vi "While_Factorial.vi"() -> ()   [LabVIEW 2024]
panel:
  out "Numeric 2":i32
  in  "Numeric":dbl
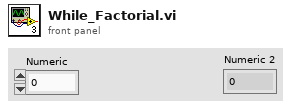
[diagram p1: front panel]
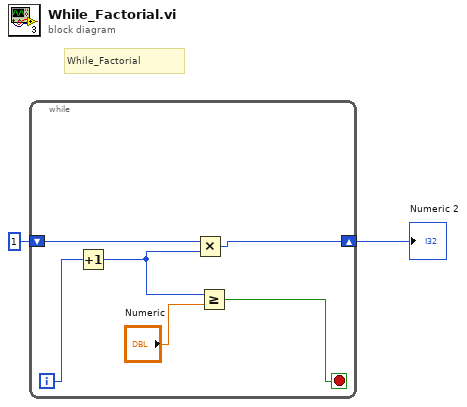
[diagram p0: block diagram]
diagram:
  # "While_Factorial"
  n1 = while {
    shift-right: [w6] -> w2
    shift-left: 1 -> [w3]
    i -> [w5]
    stop <- w8 stop-if-true
    n2 = Increment(x=w5) -> (x+1=w4:i32)
    n3 = Multiply(x=w3, y=w4) -> (x*y=w6:i32)
    n4 = Greater Or Equal?(x=w4, y="Numeric") -> (x >= y?=w8:bool)
  }
  "Numeric 2" <- w2
